vi "Generic command handler.vi"(8 "error in (no error)":errorcluster, 10 "Message in":refnum<class "GenericMessage.lvclass">, 11 "ConfocalStage in":refnum<class "ConfocalStage.lvclass">) -> (0 "error out":errorcluster, 2 "value":string, 3 "ConfocalStage out":refnum<class "ConfocalStage.lvclass">)   [LabVIEW 2012, in "ConfocalStage.lvclass"]
doc: "The generic_command_handler processes the command 'generic'. Commands which are not part of the predefined list of commands fall under the 'generic' command for special activity."
uses:
  ConfocalStage.lvclass
  <vilib>/Distrio/Murmex/GenericMessage/GenericMessage.lvclass
  <vilib>/Distrio/Murmex/Murmex/Murmex.lvclass
  ConfocalStage.lvclass/ConfocalStage.ctl
  <vilib>/Distrio/Murmex/Message/Message.lvclass
panel:
  # "This method is called when the GENERIC\ntrigger is sent. \n\nOverride this method when your component needs to\nrespond to this trigger. \n\nCall parent for proper implementation"
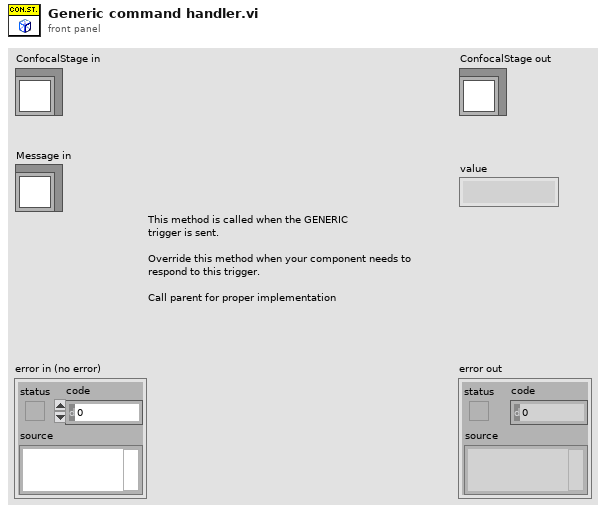
[diagram p1: front panel]
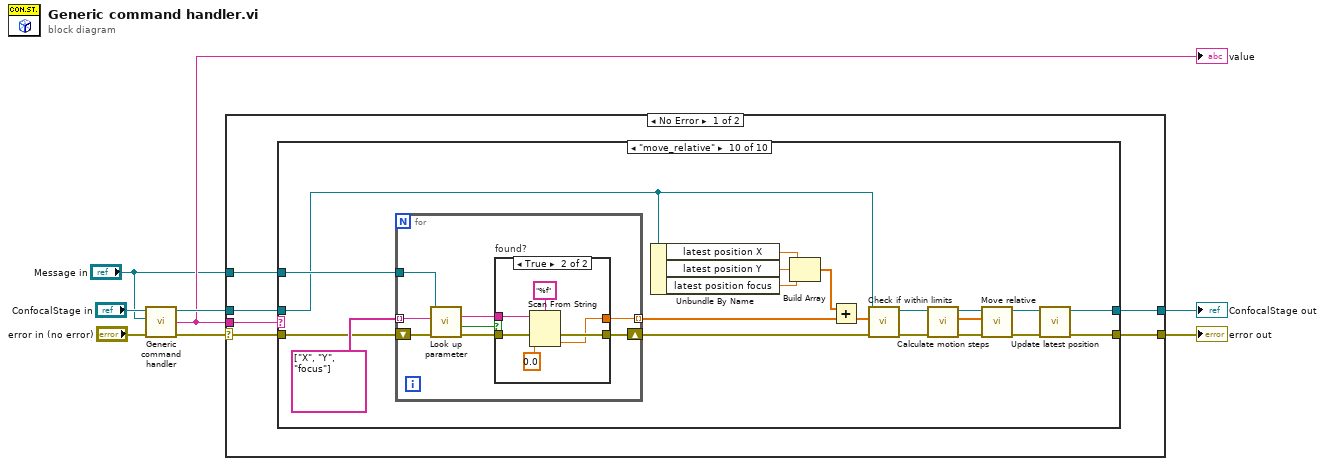
[diagram p0: block diagram]
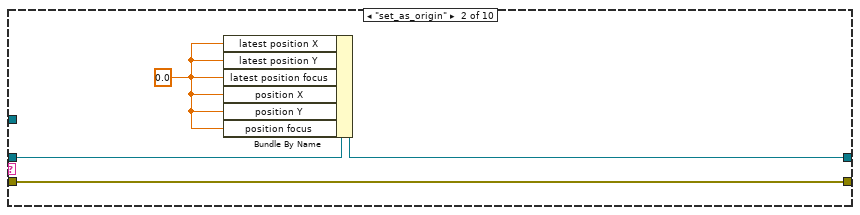
[diagram p3: hidden frame]
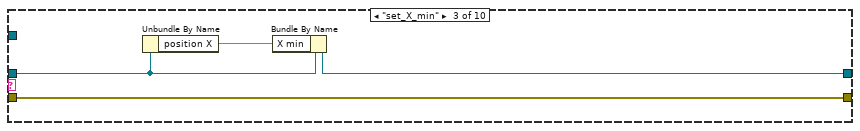
[diagram p4: hidden frame]
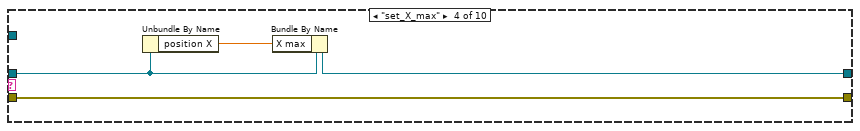
[diagram p5: hidden frame]
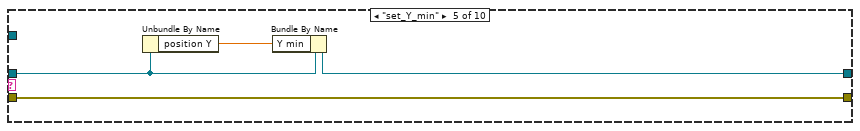
[diagram p6: hidden frame]
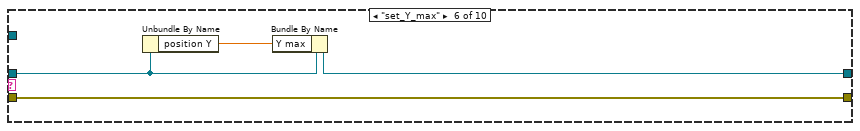
[diagram p7: hidden frame]
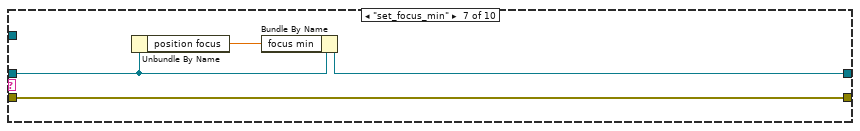
[diagram p8: hidden frame]
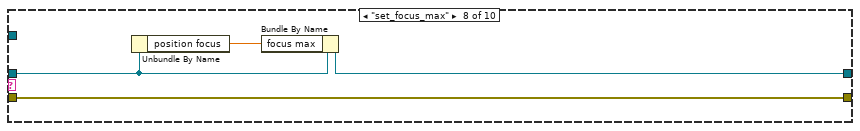
[diagram p9: hidden frame]
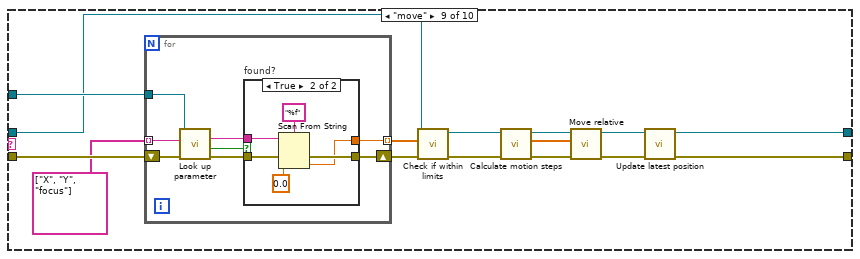
[diagram p10: hidden frame]
diagram:
  n1 = call-parent "Generic command handler.vi"("error in (no error)"="error in (no error)", "Message in"="Message in", "Murmex in"="ConfocalStage in") -> ("error out"=w6:errorcluster, "value"=w2:string, "Murmex out"=w5:refnum<class "ConfocalStage.lvclass">)  [unwired: 6 in]
  "value" <- w2
  n2 = case shown="No Error" w6 {
    selector: w6 -> [w12 w110]
    tunnel: w5 -> [w10 w111]
    tunnel: [w11 w111] -> w4
    tunnel: [w13 w110] -> w3
    tunnel: w2 -> [w14 _]
    tunnel: "Message in" -> [w9 _]
    frame No Error {
      n3 = case shown="\"move_relative\"" w14 {
        tunnel: [w16 w18 w21 w25 w29 w33 w37 w41 w45 w75] -> w13
        tunnel: w12 -> [w16 w18 w21 w25 w29 w33 w37 w41 w59 w85]
        tunnel: [w15 w19 w23 w27 w31 w35 w39 w43 w46 w76] -> w11
        tunnel: w10 -> [w15 w20 w24 w28 w32 w36 w40 w44 w54 w83]
        tunnel: w9 -> [_ _ _ _ _ _ _ _ w58 w84]
        frame Default {
        }
        frame "set_as_origin" {
          w17 = 0.0 ("runtime.position X")
          n4 = Bundle By Name(cluster=w20, "latest position X"=w17, "latest position Y"=w17, "latest position focus"=w17, "position X"=w17, "position Y"=w17, "position focus"=w17) -> (w19:refnum<class "ConfocalStage.lvclass">)
        }
        frame "set_X_min" {
          n5 = Unbundle By Name(w24) -> ("position X"=w22:dbl)
          n6 = Bundle By Name(cluster=w24, "X min"=w22) -> (w23:refnum<class "ConfocalStage.lvclass">)
        }
        frame "set_X_max" {
          n7 = Unbundle By Name(w28) -> ("position X"=w26:dbl)
          n8 = Bundle By Name(cluster=w28, "X max"=w26) -> (w27:refnum<class "ConfocalStage.lvclass">)
        }
        frame "set_Y_min" {
          n9 = Unbundle By Name(w32) -> ("position Y"=w30:dbl)
          n10 = Bundle By Name(cluster=w32, "Y min"=w30) -> (w31:refnum<class "ConfocalStage.lvclass">)
        }
        frame "set_Y_max" {
          n11 = Unbundle By Name(w36) -> ("position Y"=w34:dbl)
          n12 = Bundle By Name(cluster=w36, "Y max"=w34) -> (w35:refnum<class "ConfocalStage.lvclass">)
        }
        frame "set_focus_min" {
          n13 = Unbundle By Name(w40) -> ("position focus"=w38:dbl)
          n14 = Bundle By Name(cluster=w40, "focus min"=w38) -> (w39:refnum<class "ConfocalStage.lvclass">)
        }
        frame "set_focus_max" {
          n15 = Unbundle By Name(w44) -> ("position focus"=w42:dbl)
          n16 = Bundle By Name(cluster=w44, "focus max"=w42) -> (w43:refnum<class "ConfocalStage.lvclass">)
        }
        frame "move" {
          n17 = for {
            tunnel: w58 -> [w63]
            shift-right: [w62] -> w56
            shift-left: w59 -> [w64]
            tunnel: string[] ["X", "Y", "focus"] -> [w61] mode=indexing
            tunnel: [w60] -> w55 mode=indexing
            n18 = call <vilib>:"Look up parameter.vi"("error in (no error)"=w64, "name"=w61, "Message in"=w63) -> ("error out"=w66:errorcluster, "found?"=w67:bool, "key"=w65:string)  [unwired: 5 in, 1 out]
            n19 = case "found?" shown="True" w67 {
              tunnel: w66 -> [w68 w73]
              tunnel: w65 -> [_ w72]
              tunnel: [w68 w70] -> w62
              tunnel: [_ w69] -> w60
              frame False {
              }
              frame True {
                n20 = Scan From String(format string="%f", input string=w72, error in=w73, default 1=0.0 ("default value 1")) -> (error out=w70:errorcluster, output 1=w69:dbl)  [unwired: 1 in, 2 out]
              }
            }
          }
          n21 = call-dynamic "Check if within limits.vi"("error in (no error)"=w56, "Target position array"=w55, "ConfocalStage in"=w54) -> ("error out"=w52:errorcluster, "ConfocalStage out"=w53:refnum<class "ConfocalStage.lvclass">)  [unwired: 6 in, 1 out]
          n22 = call-dynamic "Calculate motion steps.vi"("error in (no error)"=w52, "ConfocalStage in"=w53) -> ("error out"=w49:errorcluster, "Relative motion array"=w50:dbl[], "ConfocalStage out"=w51:refnum<class "ConfocalStage.lvclass">)  [unwired: 7 in]
          n23 = call-dynamic "Move relative.vi"("error in (no error)"=w49, "Move array"=w50, "ConfocalStage in"=w51) -> ("error out"=w48:errorcluster, "ConfocalStage out"=w47:refnum<class "ConfocalStage.lvclass">)  [unwired: 7 in]
          n24 = call-dynamic "Update latest position.vi"("error in (no error)"=w48, "ConfocalStage in"=w47) -> ("error out"=w45:errorcluster, "ConfocalStage out"=w46:refnum<class "ConfocalStage.lvclass">)  [unwired: 8 in]
        }
        frame "move_relative" {
          n25 = for {
            tunnel: w84 -> [w98]
            shift-right: [w97] -> w93
            shift-left: w85 -> [w99]
            tunnel: string[] ["X", "Y", "focus"] -> [w96] mode=indexing
            tunnel: [w95] -> w79 mode=indexing
            n26 = call <vilib>:"Look up parameter.vi"("error in (no error)"=w99, "name"=w96, "Message in"=w98) -> ("error out"=w101:errorcluster, "found?"=w102:bool, "key"=w100:string)  [unwired: 5 in, 1 out]
            n27 = case "found?" shown="True" w102 {
              tunnel: w101 -> [w103 w108]
              tunnel: w100 -> [_ w107]
              tunnel: [w103 w105] -> w97
              tunnel: [_ w104] -> w95
              frame False {
              }
              frame True {
                n28 = Scan From String(format string="%f", input string=w107, error in=w108, default 1=0.0 ("default value 1")) -> (error out=w105:errorcluster, output 1=w104:dbl)  [unwired: 1 in, 2 out]
              }
            }
          }
          n29 = Unbundle By Name(w83) -> ("latest position X"=w81:dbl, "latest position Y"=w82:dbl, "latest position focus"=w80:dbl)
          n30 = Build Array(w81, w82, w80) -> (w78:dbl[])
          n31 = Add(x=w78, y=w79) -> (x+y=w77:dbl[])
          n32 = call-dynamic "Check if within limits.vi"("error in (no error)"=w93, "Target position array"=w77, "ConfocalStage in"=w83) -> ("error out"=w91:errorcluster, "ConfocalStage out"=w92:refnum<class "ConfocalStage.lvclass">)  [unwired: 6 in, 1 out]
          n33 = call-dynamic "Calculate motion steps.vi"("error in (no error)"=w91, "ConfocalStage in"=w92) -> ("error out"=w88:errorcluster, "Relative motion array"=w89:dbl[], "ConfocalStage out"=w90:refnum<class "ConfocalStage.lvclass">)  [unwired: 7 in]
          n34 = call-dynamic "Move relative.vi"("error in (no error)"=w88, "Move array"=w89, "ConfocalStage in"=w90) -> ("error out"=w87:errorcluster, "ConfocalStage out"=w86:refnum<class "ConfocalStage.lvclass">)  [unwired: 7 in]
          n35 = call-dynamic "Update latest position.vi"("error in (no error)"=w87, "ConfocalStage in"=w86) -> ("error out"=w75:errorcluster, "ConfocalStage out"=w76:refnum<class "ConfocalStage.lvclass">)  [unwired: 8 in]
        }
      }
    }
    frame Error {
    }
  }
  "error out" <- w3
  "ConfocalStage out" <- w4
